vi "ProyectoBioCuinique Beta 1.1.vi"() -> ()   [LabVIEW 2019]
uses:
  <vilib>/Utility/NIReport.llb/Report Type.ctl
  <extravilib>/ChannelInstances/Tag-dbl/Read With Abort.vi
  <extravilib>/ChannelInstances/Tag-bool/Read With Abort.vi
  <extravilib>/ChannelInstances/Tag-bool/Write With Abort.vi
  <extravilib>/ChannelInstances/Tag-dbl/Write With Abort.vi
  <vilib>/Instr/_visa.llb/VISA Configure Serial Port (Instr).vi
  <vilib>/MakerHub/LINX/Public/Utilities/Open Serial.vi
  <extravilib>/ChannelInstances/Tag-dbl/Instantiate.vi
  <extravilib>/ChannelInstances/Tag-bool/Instantiate.vi
  <extravilib>/ChannelInstances/Tag-dbl/EndpointRead.vi
  <vilib>/addons/_office/excel.llb/Excel Easy Table (str).vi
  <extravilib>/ChannelInstances/Tag-bool/EndpointRead.vi
  <extravilib>/ChannelInstances/Tag-bool/Endpoint.vi
  <extravilib>/ChannelInstances/Tag-dbl/Endpoint.vi
  <vilib>/Utility/NIReport.llb/NI_report.lvclass
  <vilib>/LabVIEW Interface for Arduino/LabVIEW Interface for Arduino.lvlib
  <vilib>/MakerHub/LINX/LMH-LINX.lvlib
  <vilib>/Utility/NIReport.llb/NI_ReportGenerationCore.lvlib
  <vilib>/addons/_office/NI_ReportGenerationToolkit.lvlib
  <vilib>/Utility/NIReport.llb/Excel/NI_Excel.lvclass
  <vilib>/MakerHub/LINX/Public/Sensors/Distance/Ultrasonic/Ultrasonic.lvlib
  <extravilib>/ChannelInstances/Tag-bool.lvlib
  <extravilib>/ChannelInstances/Tag-dbl.lvlib
panel:
  out "Hs2 4":dbl(knob) scale=0.0..100.0
  out "C° 4":dbl(slide) scale=0.0..50.0
  out "?":dbl
  out "?":dbl
  out "?":dbl
  out "Hr1 4":dbl(knob) scale=0.0..100.0
  out "Hs2 3":dbl(knob) scale=0.0..100.0
  out "C° 3":dbl(slide) scale=0.0..50.0
  out "?":dbl
  out "?":dbl
  out "?":dbl
  out "Hr1 3":dbl(knob) scale=0.0..100.0
  out "Hs2 2":dbl(knob) scale=0.0..100.0
  out "C° 2":dbl(slide) scale=0.0..50.0
  out "?":dbl
  out "?":dbl
  out "?":dbl
  out "Hr1 2":dbl(knob) scale=0.0..100.0
  out "cm 2":dbl
  out "Nivel de Agua 2":dbl(slide) scale=0.0..275.0
  out "Nivel de Agua":dbl(slide) scale=0.0..275.0
  in  "?":u8
  in  "?":u8
  in  "?":u8
  out "?":bool
  in  "?":bool
  out "?":bool
  in  "?":bool
  out "?":bool
  out "Hs2":dbl(knob) scale=0.0..100.0
  out "C°":dbl(slide) scale=0.0..50.0
  out "?":dbl
  in  "ARDUINO\nDE SENSORES\nULTRASÓNICOS":refnum<visa-resource-name>="N/A"
  in  "DATOS \n      DE  REGISTRO":path
  in  "?":u8
  in  "?":u8
  in  "?":u8
  out "?":dbl
  in  "ARDUINO DE \nSENSORES Y HUMEDAD \nY TEMPERATURA":refnum<visa-resource-name>
  out "?":dbl
  out "Hr1":dbl(knob) scale=0.0..100.0
  out "cm":dbl
  out "?":bool
  in  "?":bool
  out "?":bool
  in  "?":bool
  out "?":bool
  in  "?":bool
  in  "ARDUINO DE \nVÁLVULAS":refnum<visa-resource-name>
  # "BOMBA 1"
  # "VÁLVULA 1"
  # "VÁLVULA 2"
  # "VÁLVULA 3"
  # "BOMBA 2"
  # "VÁLVULA 4"
  # "SENSOR LINEA 2"
  # "SENSOR LINEA 4"
  # "SENSOR LINEA 1"
  # "SENSOR LINEA 3"
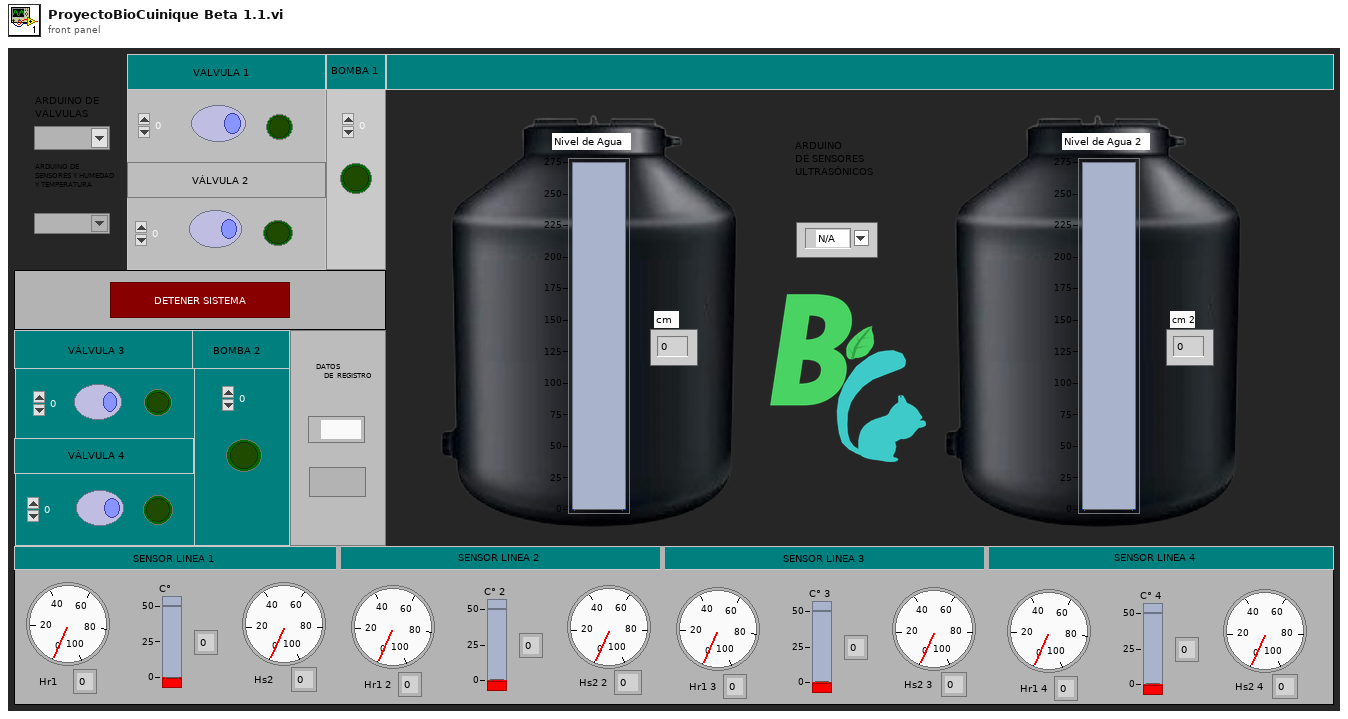
[diagram p1: front panel]
types:
  T1 = typedef "NI_ReportGenerationCore.lvlib/Report Type.ctl" = enum16{"HTML", "Word", "Excel"}
  T2 = typedef "LabVIEW Interface for Arduino.lvlib/Arduino Resource.ctl" = cluster{"VISA resource":refnum<visa-resource-name>, "Board Type":T3, "Connection Type":enum8{"USB / Serial"}, "Bytes Per Packet (15)":u8}
  T3 = typedef "LabVIEW Interface for Arduino.lvlib/Board Type.ctl" = enum16{"Uno", "Dimuelanove w/Atmega 328", "Mega 2560"}
  T4 = typedef "LMH-LINX.lvlib/LINX Ref.ctl" = cluster{"IO":T5, "Interface":T6, "LINX Device Config":T7}
  T5 = typedef "LMH-LINX.lvlib/Platform.ctl" = enum16{"Remote", "Local"}
  T6 = typedef "LMH-LINX.lvlib/Interface.ctl" = enum16{"Serial", "TCP"}
  T7 = typedef "LMH-LINX.lvlib/Device.lvlib/LINX Device Config.ctl" = cluster{"Interface":T6, "COM Port":refnum<visa-resource-name>, "TCP Configuration":T8, "Device Family":u8, "Device ID":u8, "Device Name":string, "TCP Ref":refnum<k5>, "Channels":T9}
  T8 = typedef "LMH-LINX.lvlib/Device.lvlib/TCP Config.ctl" = cluster{"IP Address":string, "Port":u16}
  T9 = typedef "LMH-LINX.lvlib/Channels.ctl" = cluster{"DI":u8[], "DO":u8[], "AI":u8[], "AO":u8[], "PWM":u8[], "QE":u8[], "UART":u8[], "I2C 2":u8[], "SPI":u8[], "CAN":u8[], "Servo":u8[], "AI Ref (V)":dbl, "AI Resolution (Bits)":u8, "AO Ref (V)":dbl, "AO Resolution (Bits)":u8}
  T10 = typedef "Tag-dbl.lvlib/))Channel.ctl" = refnum<queue>
  T11 = typedef "Tag-bool.lvlib/))Channel.ctl" = refnum<queue>
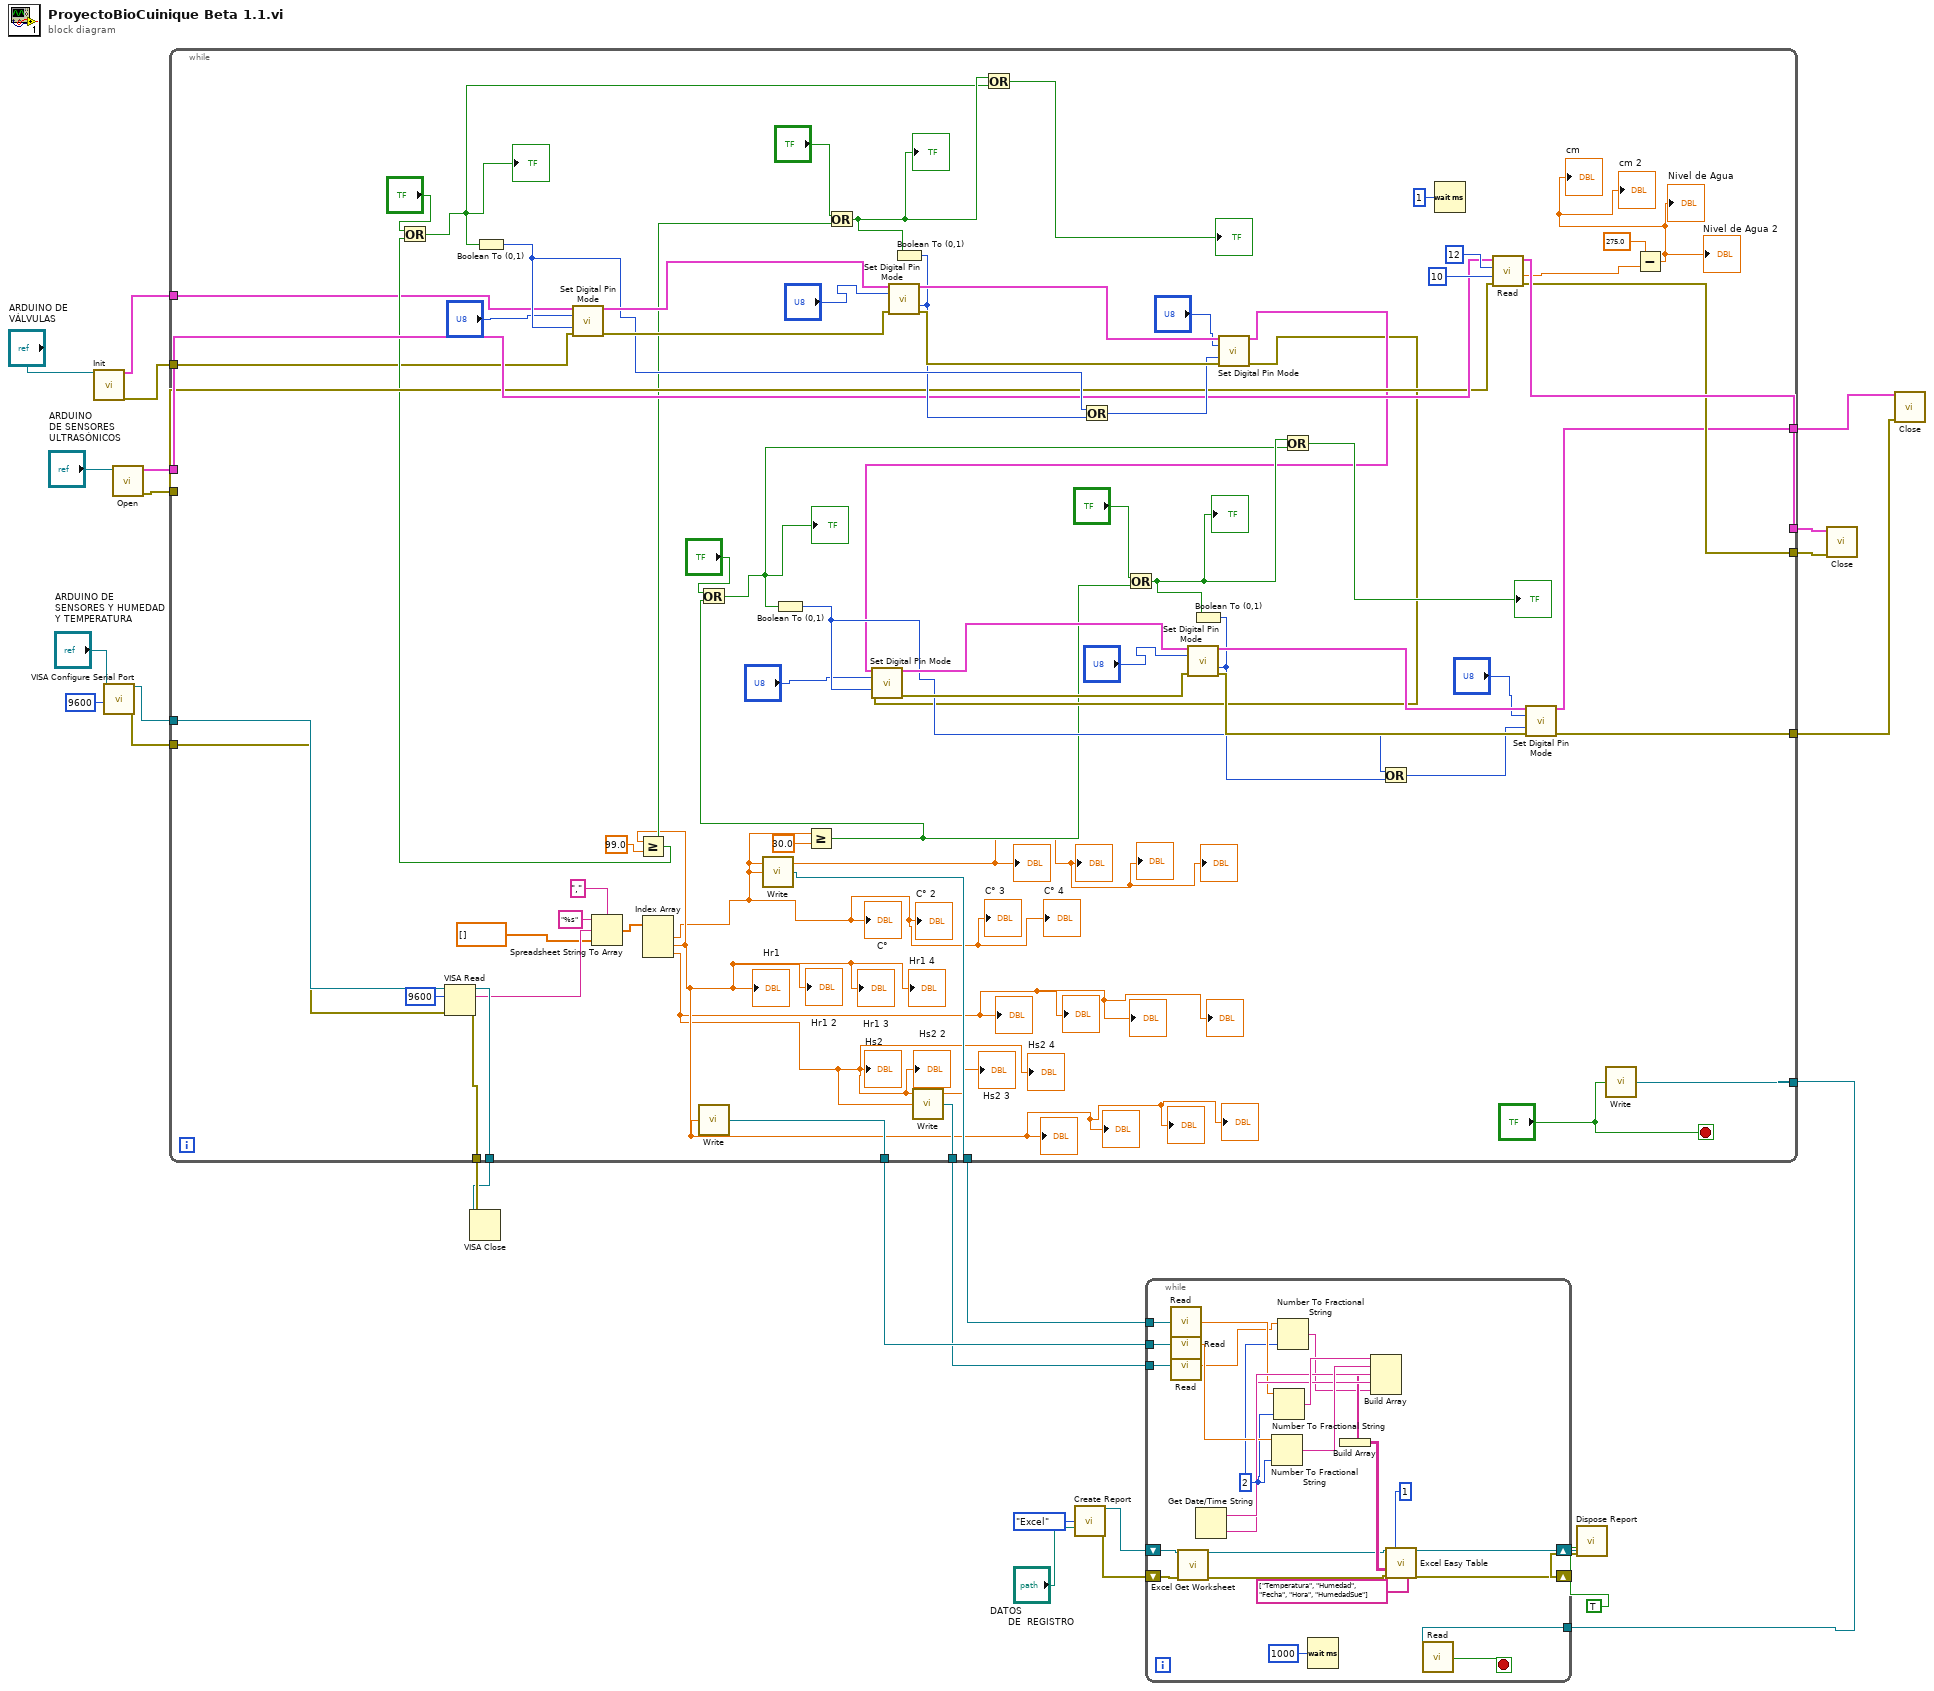
[diagram p0: block diagram]
diagram:
  n1 = call <vilib>:"Init.vi"("VISA resource"="ARDUINO DE \nVÁLVULAS") -> ("Arduino Resource"=w4:T2, "error out"=w3:errorcluster)  [unwired: 17 in]
  n2 = call-poly "VISA Configure Serial Port"("VISA resource name"="ARDUINO DE \nSENSORES Y HUMEDAD \nY TEMPERATURA", "baud rate (9600)"=u32 9600) -> ("VISA resource name out"=w22:refnum<visa-resource-name>, "error out"=w19:errorcluster)  [unwired: 12 in]
  n3 = call-poly <vilib>:"Open.vi"("Serial Port"="ARDUINO\nDE SENSORES\nULTRASÓNICOS") -> ("Error Out"=w26:errorcluster, "LINX Resource"=w25:T4)  [unwired: 8 in, 1 out]
  n4 = while {
    tunnel: w26 -> [w83]
    tunnel: w25 -> [w84]
    tunnel: [w82] -> w24
    tunnel: [w81] -> w23
    tunnel: w22 -> [w80]
    tunnel: [w79] -> w21
    tunnel: [w78] -> w20
    tunnel: w19 -> [w77]
    tunnel: [w63] -> w9
    tunnel: [w62] -> w8
    tunnel: [w61] -> w7
    tunnel: [w57] -> w5
    tunnel: w4 -> [w36]
    tunnel: w3 -> [w35]
    tunnel: [w34] -> w2
    tunnel: [w33] -> w1
    stop <- "?" stop-if-true
    n5 = VISA Read(VISA resource name=w80, byte count=u32 9600, error in (no error)=w77) -> (VISA resource name out=w78:refnum<visa-resource-name>, read buffer=w76:string, error out=w79:errorcluster)  [unwired: 1 out]
    n6 = Spreadsheet String To Array(delimiter (Tab)=",", format string="%s", spreadsheet string=w76, array type (2D Dbl)=dbl[] []) -> (array=w72:dbl[])
    n7 = Index Array(array=w72) -> (element #1=w28:dbl, element #2=w30:dbl, element #3=w29:dbl)  [unwired: 3 in]
    "Hr1" <- w30
    "?" <- w28
    "?" <- w30
    "?" <- w29
    "C°" <- w28
    "Hs2" <- w29
    "?" <- w28
    "?" <- w30
    "?" <- w29
    "C° 3" <- w28
    "Hs2 3" <- w29
    "C° 2" <- w28
    "C° 4" <- w28
    "Hs2 4" <- w29
    "Hs2 2" <- w29
    "Hr1 2" <- w30
    "Hr1 3" <- w30
    "Hr1 4" <- w30
    "?" <- w30
    "?" <- w30
    "?" <- w28
    "?" <- w28
    "?" <- w29
    "?" <- w29
    n8 = Greater Or Equal?(x=w30, y=99.0) -> (x >= y?=w60:bool)
    n9 = Or(x="?", y=w60) -> (x .or. y?=w58:bool)
    "?" <- w58
    n10 = Boolean To (0,1)(Boolean=w58) -> (0, 1=w91:i16)
    n11 = call <vilib>:"Set Digital Pin Mode.vi"("Arduino Resource"=w36, "Digital I/O Pin"="?", "Pin Mode (Input)"=w91, "error in"=w35) -> ("Arduino Resource"=w95:T2, "error out"=w94:errorcluster)  [unwired: 10 in]
    n12 = call <extravilib>:"Write.vi"("element"=w30) -> ("channel"=w61:T10)  [unwired: 1 out]
    n13 = call <extravilib>:"Write.vi"("element"=w28) -> ("channel"=w62:T10)  [unwired: 1 out]
    n14 = Greater Or Equal?(x=w28, y=30.0) -> (x >= y?=w38:bool)
    n15 = Or(x="?", y=w38) -> (x .or. y?=w42:bool)
    "?" <- w42
    n16 = Boolean To (0,1)(Boolean=w42) -> (0, 1=w52:i16)
    n17 = Or(x="?", y=w60) -> (x .or. y?=w68:bool)
    "?" <- w68
    n18 = Boolean To (0,1)(Boolean=w68) -> (0, 1=w90:i16)
    n19 = call <vilib>:"Set Digital Pin Mode.vi"("Arduino Resource"=w95, "Digital I/O Pin"="?", "Pin Mode (Input)"=w90, "error in"=w94) -> ("Arduino Resource"=w92:T2, "error out"=w93:errorcluster)  [unwired: 10 in]
    n20 = call <extravilib>:"Write.vi"("element"=w29) -> ("channel"=w57:T10)  [unwired: 1 out]
    n21 = Or(x=w68, y=w58) -> (x .or. y?=→"?":bool)
    n22 = Or(x=w91, y=w90) -> (x .or. y?=w89:i16)
    n23 = Or(x="?", y=w38) -> (x .or. y?=w47:bool)
    "?" <- w47
    n24 = Boolean To (0,1)(Boolean=w47) -> (0, 1=w51:i16)
    n25 = call <vilib>:"Set Digital Pin Mode.vi"("Arduino Resource"=w92, "Digital I/O Pin"="?", "Pin Mode (Input)"=w89, "error in"=w93) -> ("Arduino Resource"=w41:T2, "error out"=w40:errorcluster)  [unwired: 10 in]
    n26 = call <vilib>:"Set Digital Pin Mode.vi"("Arduino Resource"=w41, "Digital I/O Pin"="?", "Pin Mode (Input)"=w52, "error in"=w40) -> ("Arduino Resource"=w56:T2, "error out"=w55:errorcluster)  [unwired: 10 in]
    n27 = call <vilib>:"Set Digital Pin Mode.vi"("Arduino Resource"=w56, "Digital I/O Pin"="?", "Pin Mode (Input)"=w51, "error in"=w55) -> ("Arduino Resource"=w53:T2, "error out"=w54:errorcluster)  [unwired: 10 in]
    n28 = Or(x=w47, y=w42) -> (x .or. y?=→"?":bool)
    n29 = Or(x=w52, y=w51) -> (x .or. y?=w50:i16)
    n30 = Wait (ms)(milliseconds to wait=u32 1) -> ()  [unwired: 1 out]
    n31 = call <vilib>:"Read.vi"("Error In"=w83, "DO Channel"=u8 10, "DI Channel"=u8 12, "LINX Resource"=w84) -> ("Error Out"=w81:errorcluster, "Centimeters"=w32:dbl, "LINX Resource"=w82:T4)  [unwired: 4 in, 1 out]
    n32 = call <vilib>:"Set Digital Pin Mode.vi"("Arduino Resource"=w53, "Digital I/O Pin"="?", "Pin Mode (Input)"=w50, "error in"=w54) -> ("Arduino Resource"=w34:T2, "error out"=w33:errorcluster)  [unwired: 10 in]
    n33 = call <extravilib>:"Write.vi"("element"="?") -> ("channel"=w63:T11)  [unwired: 1 out]
    n34 = Subtract(x=275.0, y=w32) -> (x-y=→"cm" →"Nivel de Agua" →"Nivel de Agua 2" →"cm 2":dbl)
  }
  n35 = VISA Close(VISA resource name=w20, error in (no error)=w21) -> ()  [unwired: 1 out]
  n36 = call <vilib>:"Create Report.vi"("report type"=Report_Type."Excel", "template (empty)"="DATOS \n      DE  REGISTRO") -> ("report out"=w13:refnum<class "NI_report.lvclass">, "error out"=w14:errorcluster)  [unwired: 12 in]
  n37 = while {
    shift-right: [w109] -> w11
    shift-left: w14 -> [w114]
    shift-right: [w110] -> w12
    shift-left: w13 -> [w112]
    tunnel: w9 -> [w105]
    tunnel: w8 -> [w103]
    tunnel: w7 -> [w101]
    tunnel: w5 -> [w99]
    stop <- w104 stop-if-true
    w98 = i16 2 ("precision (6)")
    n38 = call <vilib>:"Read.vi"("channel"=w103) -> ("element"=w102:dbl)  [unwired: 1 in, 1 out]
    n39 = call <vilib>:"Read.vi"("channel"=w101) -> ("element"=w100:dbl)  [unwired: 1 in, 1 out]
    n40 = call <vilib>:"Read.vi"("channel"=w99) -> ("element"=w97:dbl)  [unwired: 1 in, 1 out]
    n41 = call <vilib>:"Excel Get Worksheet.vi"("report in"=w112, "error in (no error)"=w114) -> ("report out"=w111:refnum<class "NI_report.lvclass">, "error out"=w113:errorcluster)  [unwired: 12 in]
    n42 = Get Date/Time String() -> (date string=w118:string, time string=w117:string)  [unwired: 3 in]
    n43 = Number To Fractional String(number=w100, precision (6)=w98) -> (F-format string=w119:string)  [unwired: 2 in]
    n44 = Number To Fractional String(number=w102, precision (6)=w98) -> (F-format string=w120:string)  [unwired: 2 in]
    n45 = Number To Fractional String(number=w97, precision (6)=w98) -> (F-format string=w96:string)  [unwired: 2 in]
    n46 = Wait (ms)(milliseconds to wait=u32 1000) -> ()  [unwired: 1 out]
    n47 = Build Array(w120, w119, w118, w117, w96) -> (w116:string[])
    n48 = Build Array(w116) -> (w115:string[][])
    n49 = call-poly <vilib>:"Excel Easy Table.vi"("report in"=w111, "iteration"=1, "text data"=w115, "error in (no error)"=w113, "column headers"=string[] ["Temperatura", "Humedad", "Fecha", "Hora", "HumedadSue"]) -> ("report out"=w110:refnum<class "NI_report.lvclass">, "error out"=w109:errorcluster)  [unwired: 6 in, 3 out]
    n50 = call <vilib>:"Read.vi"("channel"=w105) -> ("element"=w104:bool)  [unwired: 1 in, 1 out]
  }
  n51 = call-dynamic "Dispose Report.vi"("report in"=w12, "save changes? (F)"=TRUE, "error in (no error)"=w11) -> ()  [unwired: 12 in, 1 out]
  n52 = call <vilib>:"Close.vi"("Error In"=w23, "LINX Resource"=w24) -> ()  [unwired: 9 in, 1 out]
  n53 = call <vilib>:"Close.vi"("Arduino Resource"=w2, "error in"=w1) -> ()  [unwired: 13 in, 1 out]
